vi "Add Multiple Headers.vi"(8 "error in":errorcluster, 10 "headers":cluster{"header":string, "value":string}[](array[cluster]), 11 "http-client in":refnum<class "http-client.lvclass">) -> (0 "error out":errorcluster, 3 "http-client out":refnum<class "http-client.lvclass">)   [LabVIEW 2025, in "http-client.lvclass"]
uses:
  http-client.lvclass
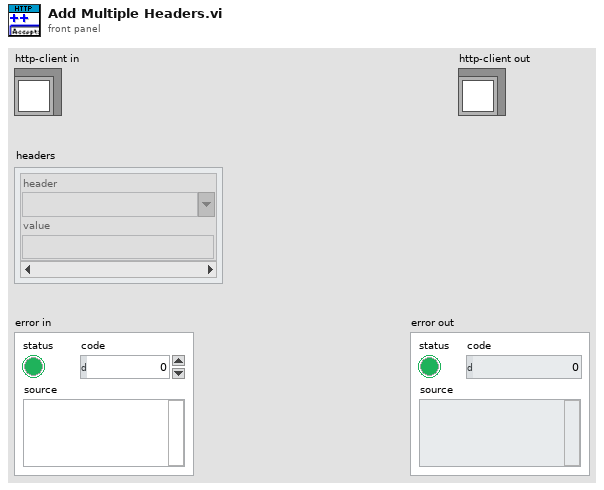
[diagram p1: front panel]
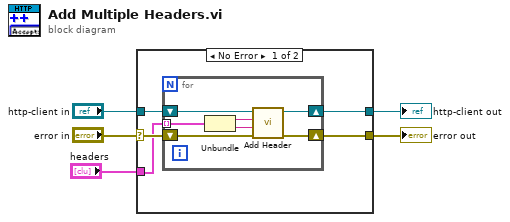
[diagram p0: block diagram]
diagram:
  n1 = case shown="No Error" "error in" {
    selector: "error in" -> [w9 w19]
    tunnel: [w7 w19] -> w4
    tunnel: [w6 w18] -> w2
    tunnel: "http-client in" -> [w10 w18]
    tunnel: "headers" -> [w8 _]
    frame No Error {
      n2 = for {
        shift-right: [w11] -> w7
        shift-left: w9 -> [w12]
        shift-right: [w15] -> w6
        shift-left: w10 -> [w16]
        tunnel: w8 -> [w17] mode=indexing
        n3 = Unbundle(w17) -> ("header"=w14:string, "value"=w13:string)
        n4 = call "Add Header.vi"("error in"=w12, "value"=w13, "header"=w14, "http-client in"=w16) -> ("error out"=w11:errorcluster, "http-client out"=w15:refnum<class "http-client.lvclass">)  [unwired: 6 in]
      }
    }
    frame Error {
    }
  }
  "error out" <- w4
  "http-client out" <- w2
